vi "ttm_tampereCyclic_poller.vi"() -> ()   [LabVIEW 2010]
panel:
  in  "sampleHeigth":dbl=-4.7
  in  "Input cluster":T1 {"Set Point" format="%.2f"; "Ramp Amplitude" format="%.2f"; "Ramp Rate" format="%.2f"; "Set Point Time" format="%.2f"}
  in  "strain":dbl[](array[numeric])
  in  "ramprate":dbl=0.02
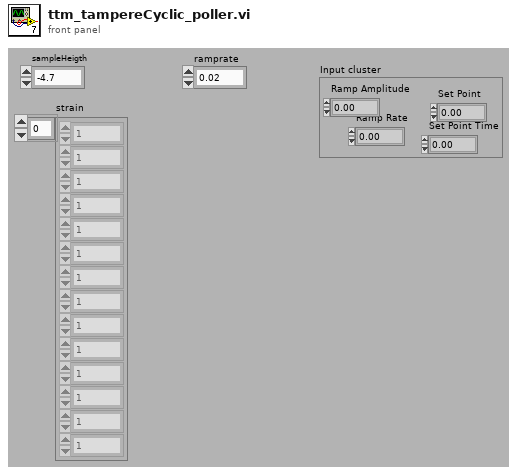
[diagram p1: front panel]
types:
  T1 = cluster{"Set Point":dbl, "Set Point Time":dbl, "Ramp Amplitude":dbl, "Ramp Rate":dbl}
  T2 = cluster{"Name":string, "Type":i32, "SI Full Scale":dbl, "Full Scale":dbl, "Units String":string, "Display Format":string, "Gauge Length":dbl}[][]
  T3 = cluster{"Device ID":i32, "Device Name":string, "Device Type":i32}[]
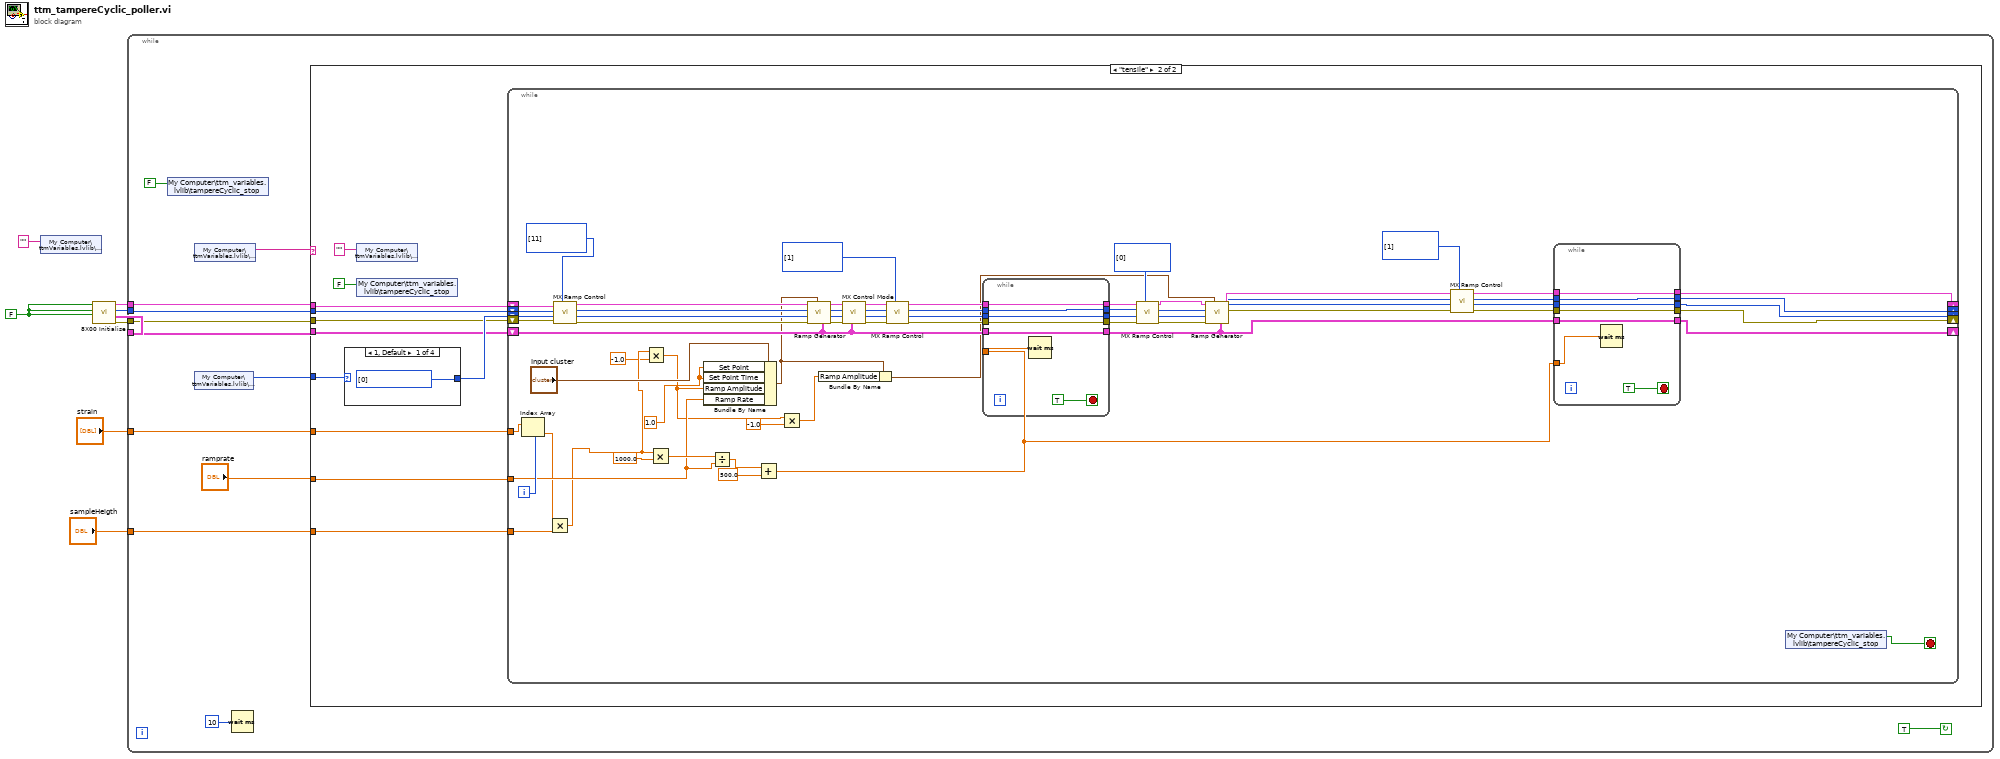
[diagram p0: block diagram]
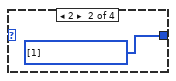
[diagram p3: hidden frame]
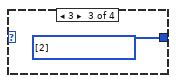
[diagram p4: hidden frame]
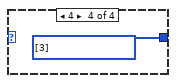
[diagram p5: hidden frame]
diagram:
  w4 = FALSE ("Reset?")
  n1 = shared-variable "My Computer\\ttmVariables.lvlib\\protocol"("" ("protocol")) -> ()  [unwired: 1 in, 1 out]
  n2 = call "8X00 Initialise.vi"("Reset?"=w4, "Create DVM? (T)"=w4, "Create Console? (T)"=w4) -> ("error out"=w5:errorcluster, "Channel Data"=w8:T2, "Axis Selector"=w6:i32[], "Axis Information"=w7:T3)  [unwired: 1 in]
  n3 = while {
    tunnel: w8 -> [w17]
    tunnel: w7 -> [w18]
    tunnel: w6 -> [w19]
    tunnel: w5 -> [w16]
    tunnel: "strain" -> [w10]
    tunnel: "sampleHeigth" -> [w9]
    stop <- TRUE continue-if-true
    n4 = shared-variable "My Computer\\ttm_variables.lvlib\\tampereCyclic_stop"(FALSE ("tampereCyclic_stop")) -> ()  [unwired: 1 in, 1 out]
    n5 = shared-variable "My Computer\\ttmVariables.lvlib\\protocol"() -> (w12:string)  [unwired: 1 in, 1 out]
    n6 = shared-variable "My Computer\\ttmVariables.lvlib\\channel"() -> (w13:i32)  [unwired: 1 in, 1 out]
    n7 = Wait (ms)(milliseconds to wait=u32 10) -> ()  [unwired: 1 out]
    n8 = case shown="\"tensile\"" w12 {
      tunnel: w19 -> [_ w30]
      tunnel: w18 -> [_ w29]
      tunnel: w17 -> [_ w25]
      tunnel: w16 -> [_ w28]
      tunnel: "ramprate" -> [_ w27]
      tunnel: w13 -> [_ w26]
      tunnel: w10 -> [_ w22]
      tunnel: w9 -> [_ w21]
      frame "", Default {
      }
      frame "tensile" {
        n9 = case shown="1, Default" w26 {
          tunnel: [w113 w114 w115 w116] -> w31
          frame 1, Default {
            w113 = u16[] [0] items=["Channel 1", "Channel 2", "Channel 3", "Channel 4"] ("Choose channel to apply\nthe setpoint")
          }
          frame 2 {
            w114 = u16[] [1] items=["Channel 1", "Channel 2", "Channel 3", "Channel 4"] ("Choose channel to apply\nthe setpoint")
          }
          frame 3 {
            w115 = u16[] [2] items=["Channel 1", "Channel 2", "Channel 3", "Channel 4"] ("Choose channel to apply\nthe setpoint")
          }
          frame 4 {
            w116 = u16[] [3] items=["Channel 1", "Channel 2", "Channel 3", "Channel 4"] ("Choose channel to apply\nthe setpoint")
          }
        }
        n10 = shared-variable "My Computer\\ttmVariables.lvlib\\protocol"("" ("protocol")) -> ()  [unwired: 1 in, 1 out]
        n11 = shared-variable "My Computer\\ttm_variables.lvlib\\tampereCyclic_stop"(FALSE ("tampereCyclic_stop")) -> ()  [unwired: 1 in, 1 out]
        n12 = while {
          tunnel: w27 -> [w54]
          shift-right: [w86] -> _
          shift-left: w29 -> [w81]
          shift-right: [w85] -> _
          shift-left: w30 -> [w80]
          shift-right: [w84] -> _
          shift-left: w31 -> [w79]
          shift-right: [w83] -> _
          shift-left: w28 -> [w78]
          shift-right: [w82] -> _
          shift-left: w25 -> [w59]
          tunnel: w22 -> [w72]
          tunnel: w21 -> [w40]
          i -> [w71]
          stop <- w95 stop-if-true
          w39 = u16[] [1] items=["Stop", "Start or continue", "Hold", "Continue", "Return ramp to set level at fixed rate", "Reserved", "Reserved", "Start Random without demand hold", "Start Random with demand hold", "Prepare Random Start without demand hold", "Prepare Random Start with demand hold", "Unslave", "Reserved", "Reserved", "Start Sample Data Playback or Resume", "Prepare for Start of Sample Data", "Reserved", "Reserved", "Resume Playback", "Start an electromechanical frame return"] ("Ramp Control")
          w77 = u16[] [11] items=["Stop", "Start or continue", "Hold", "Continue", "Return ramp to set level at fixed rate", "Reserved", "Reserved", "Start Random without demand hold", "Start Random with demand hold", "Prepare Random Start without demand hold", "Prepare Random Start with demand hold", "Unslave", "Reserved", "Reserved", "Start Sample Data Playback or Resume", "Prepare for Start of Sample Data", "Reserved", "Reserved", "Resume Playback", "Start an electromechanical frame return"] ("Ramp Control")
          w97 = u16[] [0] items=["Stop", "Start or continue", "Hold", "Continue", "Return ramp to set level at fixed rate", "Reserved", "Reserved", "Start Random without demand hold", "Start Random with demand hold", "Prepare Random Start without demand hold", "Prepare Random Start with demand hold", "Unslave", "Reserved", "Reserved", "Start Sample Data Playback or Resume", "Prepare for Start of Sample Data", "Reserved", "Reserved", "Resume Playback", "Start an electromechanical frame return"] ("Ramp Control")
          w98 = u16[] [1] items=["Stop", "Start or continue", "Hold", "Continue", "Return ramp to set level at fixed rate", "Reserved", "Reserved", "Start Random without demand hold", "Start Random with demand hold", "Prepare Random Start without demand hold", "Prepare Random Start with demand hold", "Unslave", "Reserved", "Reserved", "Start Sample Data Playback or Resume", "Prepare for Start of Sample Data", "Reserved", "Reserved", "Resume Playback", "Start an electromechanical frame return"] ("Ramp Control")
          w55 = 1.0 ("Set Point Time")
          n13 = Index Array(array=w72, index=w71) -> (element=w41:dbl)
          n14 = Multiply(x=w41, y=w40) -> (x*y=w34:dbl)
          n15 = call "MX Ramp Control.vi"("Ramp Control"=w77, "error in (no error)"=w78, "Channels In"=w79, "Axis Selector In"=w80, "Axis Information In"=w81) -> ("error out"=w58:errorcluster, "Channels Out"=w57:u16[], "Axis Selector Out"=w56:i32[], "Axis Information Out"=w65:T3)  [unwired: 2 in]
          n16 = Multiply(x=w34, y=-1.0) -> (x*y=w33:dbl)
          n17 = Multiply(x=w34, y=1000.0) -> (x*y=w67:dbl)
          n18 = Bundle By Name(cluster="Input cluster", "Set Point"=w55, "Set Point Time"=w55, "Ramp Amplitude"=w33, "Ramp Rate"=w54) -> (w53:T1)
          n19 = Divide(x=w67, y=w54) -> (x/y=w70:dbl)
          n20 = Add(x=w70, y=500.0) -> (x+y=w68:dbl)
          n21 = Multiply(x=w33, y=-1.0) -> (x*y=w52:dbl)
          n22 = call "Ramp Generator.vi"("Channel Data"=w59, "Input cluster"=w53, "error in (no error)"=w58, "Channels"=w57, "Axis Selector"=w56, "Axis Information"=w65) -> ("Error Out"=w60:errorcluster, "Channels Out"=w61:u16[], "Axis Selector Out"=w62:i32[], "Axis Information Out"=w63:T3)  [unwired: 2 in]
          n23 = Bundle By Name(cluster=w53, "Ramp Amplitude"=w52) -> (w46:T1)
          n24 = call "MX Control Mode.vi"("Channel Data"=w59, "error in (no error)"=w60, "Control Modes"=w61, "Axis Selector"=w62, "Axis Information"=w63) -> ("error out"=w73:errorcluster, "Control Modes out"=w74:u16[], "Axis Selector out"=w75:i32[], "Axis Information out"=w76:T3)  [unwired: 1 in]
          n25 = call "MX Ramp Control.vi"("Ramp Control"=w98, "error in (no error)"=w73, "Channels In"=w74, "Axis Selector In"=w75, "Axis Information In"=w76) -> ("error out"=w91:errorcluster, "Channels Out"=w92:u16[], "Axis Selector Out"=w93:i32[], "Axis Information Out"=w94:T3)  [unwired: 2 in]
          n26 = while {
            tunnel: w94 -> [w108]
            tunnel: [w108] -> w87
            tunnel: w93 -> [w112]
            tunnel: [w112] -> w88
            tunnel: w92 -> [w111]
            tunnel: [w111] -> w89
            tunnel: w91 -> [w110]
            tunnel: [w110] -> w90
            tunnel: w59 -> [w107]
            tunnel: [w107] -> w47
            tunnel: w68 -> [w106]
            stop <- TRUE stop-if-true
            n27 = Wait (ms)(milliseconds to wait=w106) -> ()  [unwired: 1 out]
          }
          n28 = call "MX Ramp Control.vi"("Ramp Control"=w97, "error in (no error)"=w90, "Channels In"=w89, "Axis Selector In"=w88, "Axis Information In"=w87) -> ("error out"=w48:errorcluster, "Channels Out"=w49:u16[], "Axis Selector Out"=w50:i32[], "Axis Information Out"=w51:T3)  [unwired: 2 in]
          n29 = call "Ramp Generator.vi"("Channel Data"=w47, "Input cluster"=w46, "error in (no error)"=w48, "Channels"=w49, "Axis Selector"=w50, "Axis Information"=w51) -> ("Error Out"=w42:errorcluster, "Channels Out"=w43:u16[], "Axis Selector Out"=w44:i32[], "Axis Information Out"=w45:T3)  [unwired: 2 in]
          n30 = call "MX Ramp Control.vi"("Ramp Control"=w39, "error in (no error)"=w42, "Channels In"=w43, "Axis Selector In"=w44, "Axis Information In"=w45) -> ("error out"=w38:errorcluster, "Channels Out"=w37:u16[], "Axis Selector Out"=w36:i32[], "Axis Information Out"=w35:T3)  [unwired: 2 in]
          n31 = while {
            tunnel: w35 -> [w105]
            tunnel: [w105] -> w86
            tunnel: w36 -> [w104]
            tunnel: [w104] -> w85
            tunnel: w37 -> [w103]
            tunnel: [w103] -> w84
            tunnel: w38 -> [w102]
            tunnel: [w102] -> w83
            tunnel: w47 -> [w100]
            tunnel: [w100] -> w82
            tunnel: w68 -> [w99]
            stop <- TRUE stop-if-true
            n32 = Wait (ms)(milliseconds to wait=w99) -> ()  [unwired: 1 out]
          }
          n33 = shared-variable "My Computer\\ttm_variables.lvlib\\tampereCyclic_stop"() -> (w95:bool)  [unwired: 1 in, 1 out]
        }
      }
    }
  }
